vi "Skale_Y_ON_OFF.vi"(8 "error in (no error)":errorcluster, 10 "PlotIdx":i32, 11 "WaveformGraph in":refnum<vi>) -> (0 "error out":errorcluster)   [LabVIEW 2014]
doc: "Ustawia widoczność skal na wykresach w zależności\nod tego, które przebiegi są widoczne"
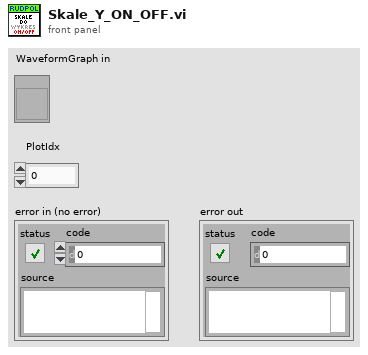
[diagram p1: front panel]
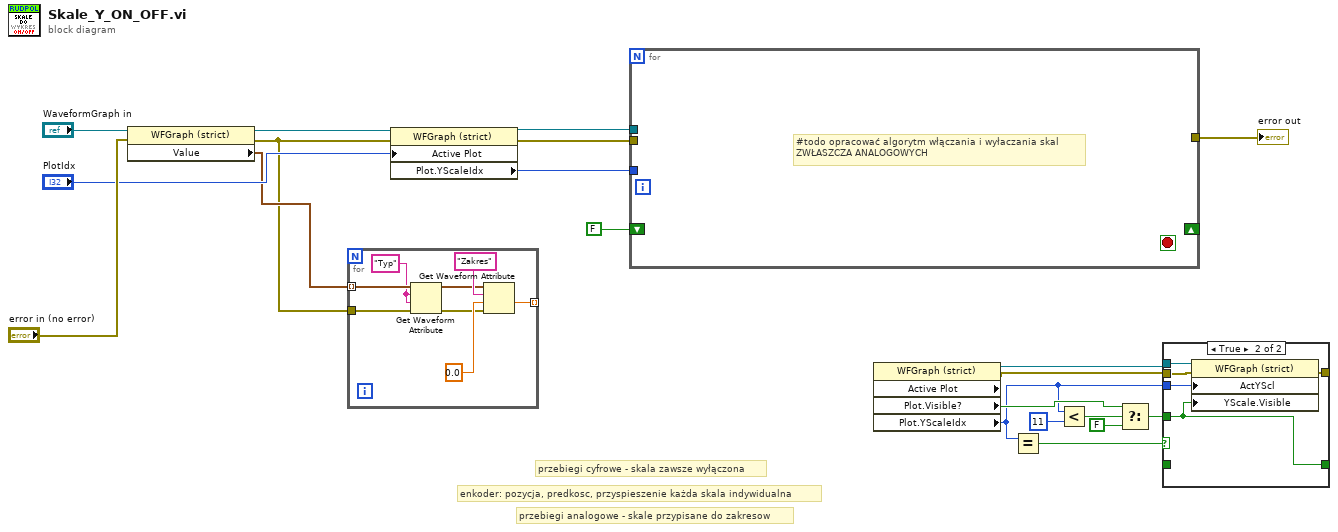
[diagram p0: block diagram]
diagram:
  # "enkoder: pozycja, predkosc, przyspieszenie każda skala indywidualna"
  # "przebiegi cyfrowe - skala zawsze wyłączona"
  # "przebiegi analogowe - skale przypisane do zakresow"
  n1 = property class="WFGraph (strict)"(reference="WaveformGraph in", error in="error in (no error)") -> (reference out=w19:refnum<vi>, error out=w15:errorcluster, "Value"=w17:waveform(dbl)[])
  n2 = for {
    tunnel: w17 -> [w30] mode=indexing
    tunnel: w15 -> [w29]
    tunnel: [w31] -> _ mode=indexing
    w28 = "Typ" ("name")
    n3 = Get Waveform Attribute(4:w29, 5:w28, 6:w28, 7:w30) -> (0:w26:errorcluster, 3:w27:waveform(dbl))  [unwired: 2 out]
    n4 = Get Waveform Attribute(4:w26, 5:0.0, 6:"Zakres" ("name"), 7:w27) -> (1:w31:dbl)  [unwired: 3 out]
  }
  n5 = property on="Property Node" class="WFGraph (strict)"(reference=w19, error in=w15, "Active Plot"="PlotIdx") -> (reference out=w21:refnum<vi>, error out=w22:errorcluster, "Plot.YScaleIdx"=w16:u32)
  n6 = for {
    tunnel: w16 -> [_]
    shift-right: _ -> [_]
    shift-left: FALSE ("Plot.Visible?") -> [_]
    tunnel: w21 -> [_]
    tunnel: w22 -> [_]
    tunnel: [_] -> w24
    stop <- _ stop-if-true
    # "#todo opracować algorytm włączania i wyłaczania skal\nZWŁASZCZA ANALOGOWYCH"
  }
  "error out" <- w24
  n7 = property on="Property Node" class="WFGraph (strict)"() -> (reference=w5:refnum<vi>, reference out=w6:refnum<vi>, error in=w8:errorcluster, error out=w7:errorcluster, "Active Plot"=w1:u32, "Plot.Visible?"=w13:bool, "Plot.YScaleIdx"=w11:u32)
  n8 = Equal?(x=w11) -> (y=w2:u32, x = y?=w3:bool)
  n9 = Less?(x=w11, y=u32 11) -> (x < y?=w10:bool)
  n10 = Select(t=w13, s=w10, f=FALSE) -> (s? t:f=w9:bool)
  n11 = case shown="True" w3 {
    tunnel: w11 -> [_ w40]
    tunnel: [w35 _] -> w4
    tunnel: [w35 w39] -> _
    tunnel: w9 -> [_ w39]
    tunnel: w6 -> [_ w38]
    tunnel: w7 -> [w34 w37]
    tunnel: [w34 w36] -> _
    frame False {
    }
    frame True {
      n12 = property on="Property Node" class="WFGraph (strict)"(reference=w38, error in=w37, "ActYScl"=w40, "YScale.Visible"=w39) -> (error out=w36:errorcluster)  [unwired: 1 out]
    }
  }
